vi "conexión arduino labview.vi"() -> ()   [LabVIEW 2020]
uses:
  <vilib>/Instr/_visa.llb/VISA Configure Serial Port (Instr).vi
panel:
  in  "OK Button":bool
  in  "stop":bool
  in  "String":string
  in  "VISA resource name":refnum<visa-resource-name>
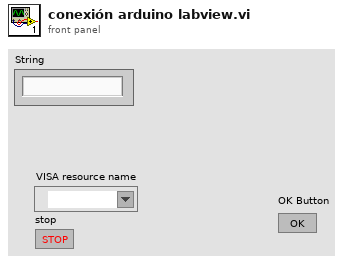
[diagram p1: front panel]
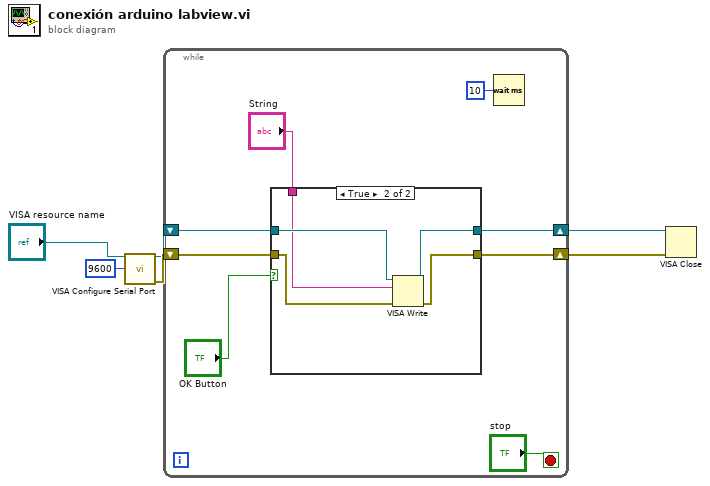
[diagram p0: block diagram]
diagram:
  n1 = call-poly "VISA Configure Serial Port"("VISA resource name"="VISA resource name", "baud rate (9600)"=u32 9600) -> ("VISA resource name out"=w1:refnum<visa-resource-name>, "error out"=w4:errorcluster)  [unwired: 12 in]
  n2 = while {
    shift-right: [w13] -> w3
    shift-left: w4 -> [w14]
    shift-right: [w12] -> w2
    shift-left: w1 -> [w11]
    stop <- "stop" stop-if-true
    n3 = case shown="True" "OK Button" {
      tunnel: w14 -> [w15 w21]
      tunnel: [w15 w20] -> w13
      tunnel: [w16 w19] -> w12
      tunnel: w11 -> [w16 w18]
      tunnel: "String" -> [_ w17]
      frame False {
      }
      frame True {
        n4 = VISA Write(VISA resource name=w18, write buffer=w17, error in (no error)=w21) -> (VISA resource name out=w19:refnum<visa-resource-name>, error out=w20:errorcluster)  [unwired: 1 out]
      }
    }
    n5 = Wait (ms)(milliseconds to wait=u32 10) -> ()  [unwired: 1 out]
  }
  n6 = VISA Close(VISA resource name=w2, error in (no error)=w3) -> ()  [unwired: 1 out]
